vi "SetROI.vi"(8 "error in (no error)":errorcluster, 10 "fullWidth?":bool, 11 "Config In":T1 {"Hardware Configuration"."Lasers Configuration"."SettingValues"."785 Power" format="%.1f"; "Hardware Configuration"."Lasers Configuration"."SettingValues"."647 Power" format="%.1f"; "Hardware Configuration"."Lasers Configuration"."SettingValues"."561 Power" format="%.1f"}) -> (0 "error out":errorcluster, 3 "Config Out":T1 {"Hardware Configuration"."Lasers Configuration"."SettingValues"."785 Power" format="%.1f"; "Hardware Configuration"."Lasers Configuration"."SettingValues"."647 Power" format="%.1f"; "Hardware Configuration"."Lasers Configuration"."SettingValues"."561 Power" format="%.1f"})   [LabVIEW 2020]
uses:
  Settings/System Running Settings.ctl
  Support/Hardware Configuration.ctl
  Support/Camera Configuration.ctl
  controls/ROI.ctl
  D:/Daguan/Development/RM21-MMicrosopeSource/HardwareAdapter/Camera/Dependencies/PVCamNET.dll
  Dependencies/PVCamNET.dll
  <vilib>/vision/Image Controls.llb/IMAQ Image.ctl
  D:/Daguan/Development/RM21-MMicrosopeSource/HardwareAdapter/Lasers/Dependencies/Oxxius_Boxx.dll
  Lasers/Dependencies/Oxxius_Boxx.dll
  Logging/Logging Configuration.ctl
  controls/DeviceStatusCtl.ctl
  controls/CallBack Refs.ctl
  Logging/Logging.lvlib
  Settings/Settings.lvlib
panel:
  in  "Full CCD Height":u16
  in  "Full CCD Width":u16
  in  "Height":u16
  in  "Y":u16
  in  "Width":u16
  in  "X":u16
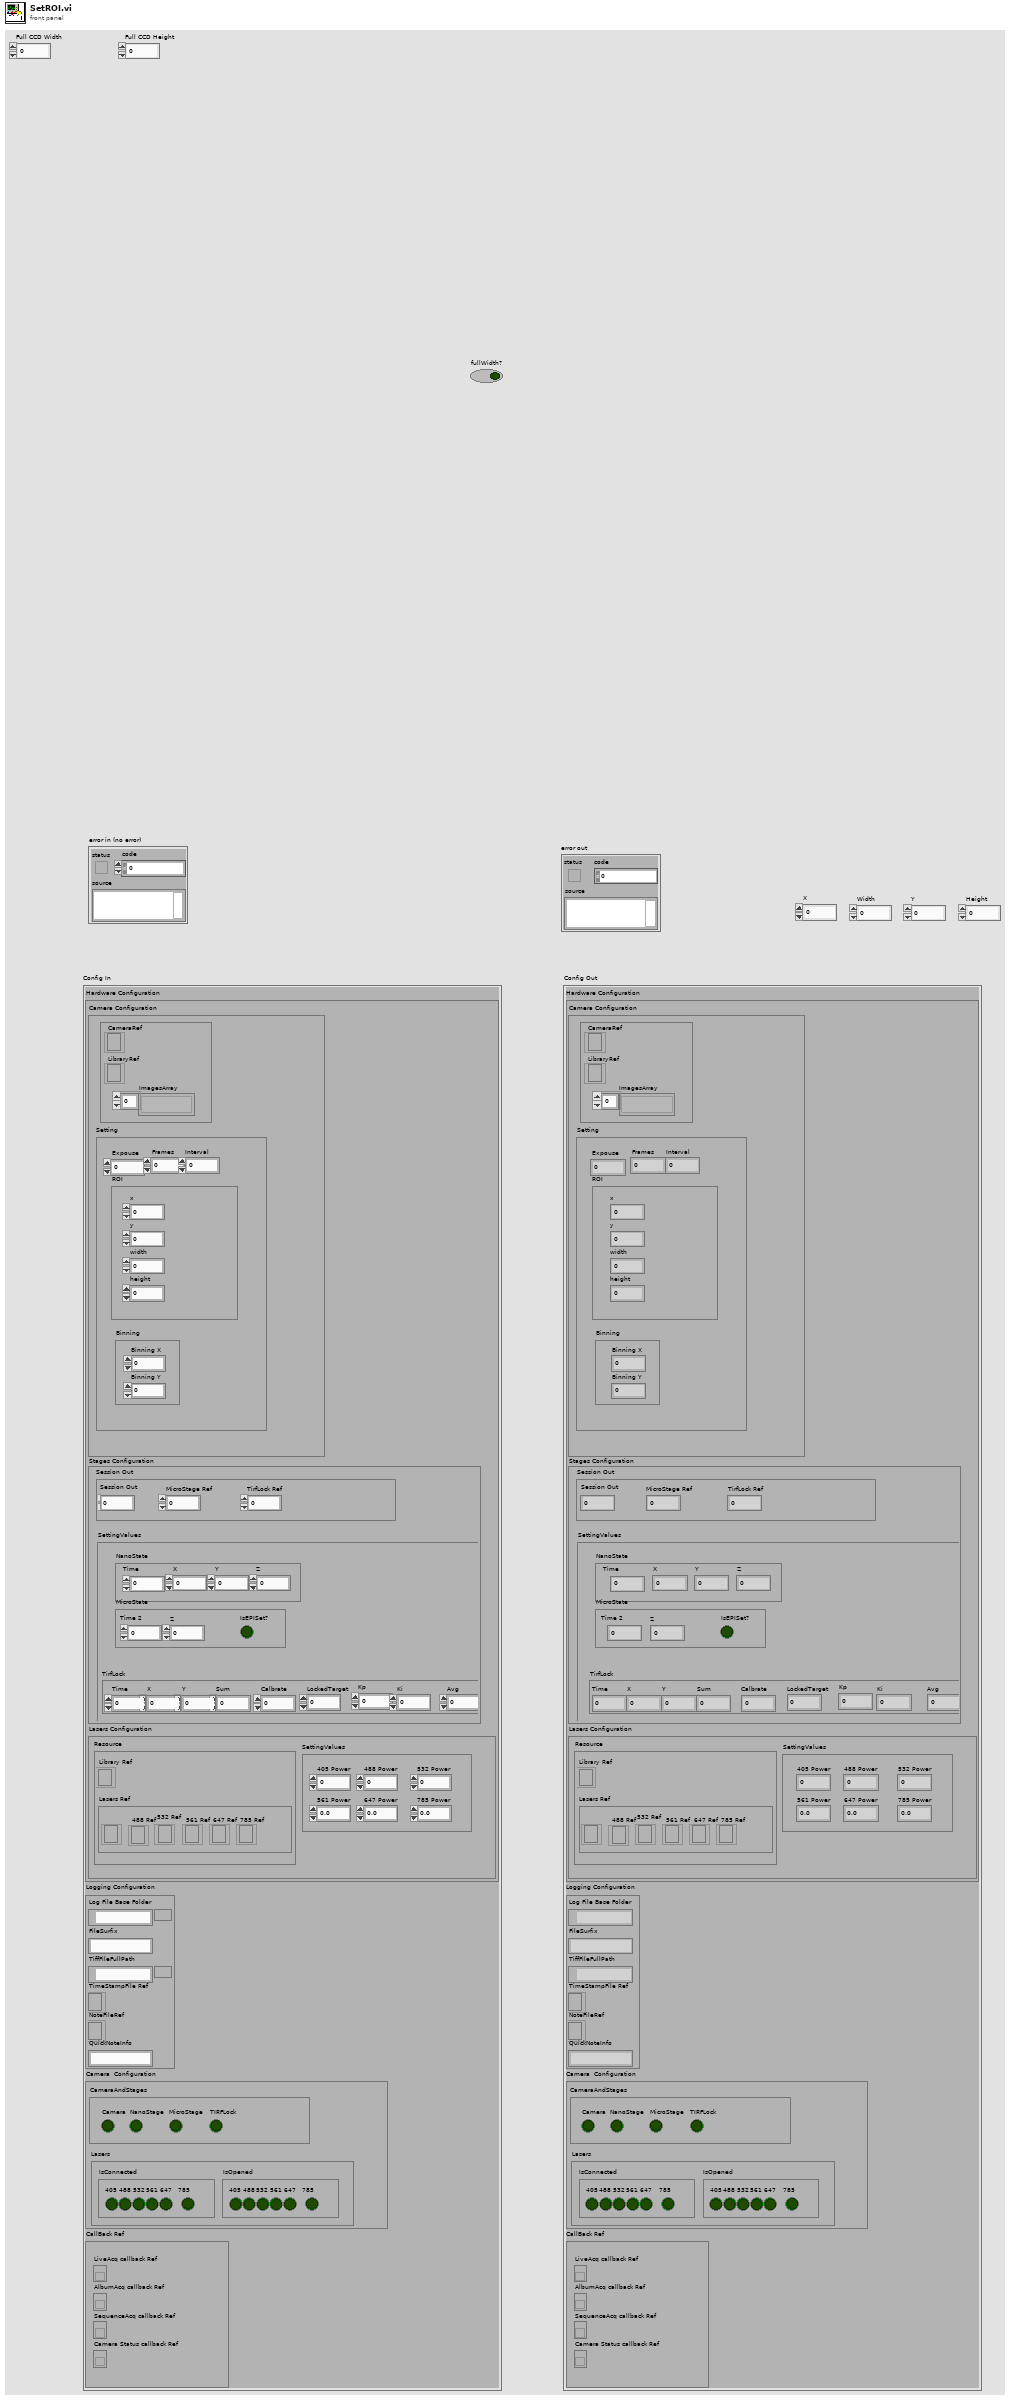
[diagram p1: front panel]
types:
  T1 = typedef "Settings.lvlib/System Running Settings.ctl" = cluster{"Hardware Configuration":T2, "Logging Configuration":T6, "HardWare Status":cluster{"CameraAndStages":T7, "Lasers":cluster{"IsConnected":cluster{"405":bool, "488":bool, "532":bool, "561":bool, "647":bool, "785":bool}, "IsOpened":cluster{"405":bool, "488":bool, "532":bool, "561":bool, "647":bool, "785":bool}}}, "CallBack Ref":T8}
  T2 = typedef "Hardware Configuration.ctl" = cluster{"Camera Configuration":T3, "Stages Configuration":cluster{"Resource":cluster{"NanoStage Ref":i32, "MicroStage Ref":i32, "TirfLock Ref":i32}, "SettingValues":cluster{"NanoState":cluster{"Time":dbl, "X":dbl, "Y":dbl, "Z":dbl}, "MicroState":cluster{"Time 2":dbl, "Z":dbl, "IsEPISet?":bool}, "TirfLock":cluster{"Time":dbl, "X":dbl, "Y":dbl, "Sum":dbl, "Calbrate":dbl, "LockedTarget":dbl, "Kp":dbl, "Ki":dbl, "Avg":dbl}}}, "Lasers Configuration":cluster{"SettingValues":cluster{"405 Power":sgl, "488 Power":sgl, "532 Power":sgl, "561 Power":sgl, "647 Power":sgl, "785 Power":sgl}, "Resource":cluster{"Library Ref":refnum<k24>, "Lasers Ref":cluster{"405 Ref":refnum<k24>, "488 Ref":refnum<k24>, "532 Ref":refnum<k24>, "561 Ref":refnum<k24>, "647 Ref":refnum<k24>, "785 Ref":refnum<k24>}}}}
  T3 = typedef "Camera Configuration.ctl" = cluster{"Setting":cluster{"Expouse":dbl, "Frames":dbl, "Interval":dbl, "ROI":T4, "Binning":cluster{"Binning X":dbl, "Binning Y":dbl}}, "Resource":cluster{"CameraRef":refnum<k24>, "LibraryRef":refnum<k24>, "ImagesArray":T5[]}}
  T4 = typedef "ROI.ctl" = cluster{"x":dbl, "y":dbl, "width":dbl, "height":dbl}
  T5 = typedef "IMAQ Image.ctl" = refnum<image>
  T6 = typedef "Logging.lvlib/Logging Configuration.ctl" = cluster{"Log File Base Folder":path, "FileSurfix":string, "TiffFileFullPath":path, "TimeStampFile Ref":refnum<file>, "NoteFileRef":refnum<file>, "QuickNoteInfo":string}
  T7 = typedef "DeviceStatusCtl.ctl" = cluster{"Camera":bool, "NanoStage":bool, "MicroStage":bool, "TIRFLock":bool}
  T8 = typedef "CallBack Refs.ctl" = cluster{"LiveAcq callback Ref":refnum<k27>, "AlbumAcq callback Ref":refnum<k27>, "SequenceAcq callback Ref":refnum<k27>, "Camera Status callback Ref":refnum<k27>}
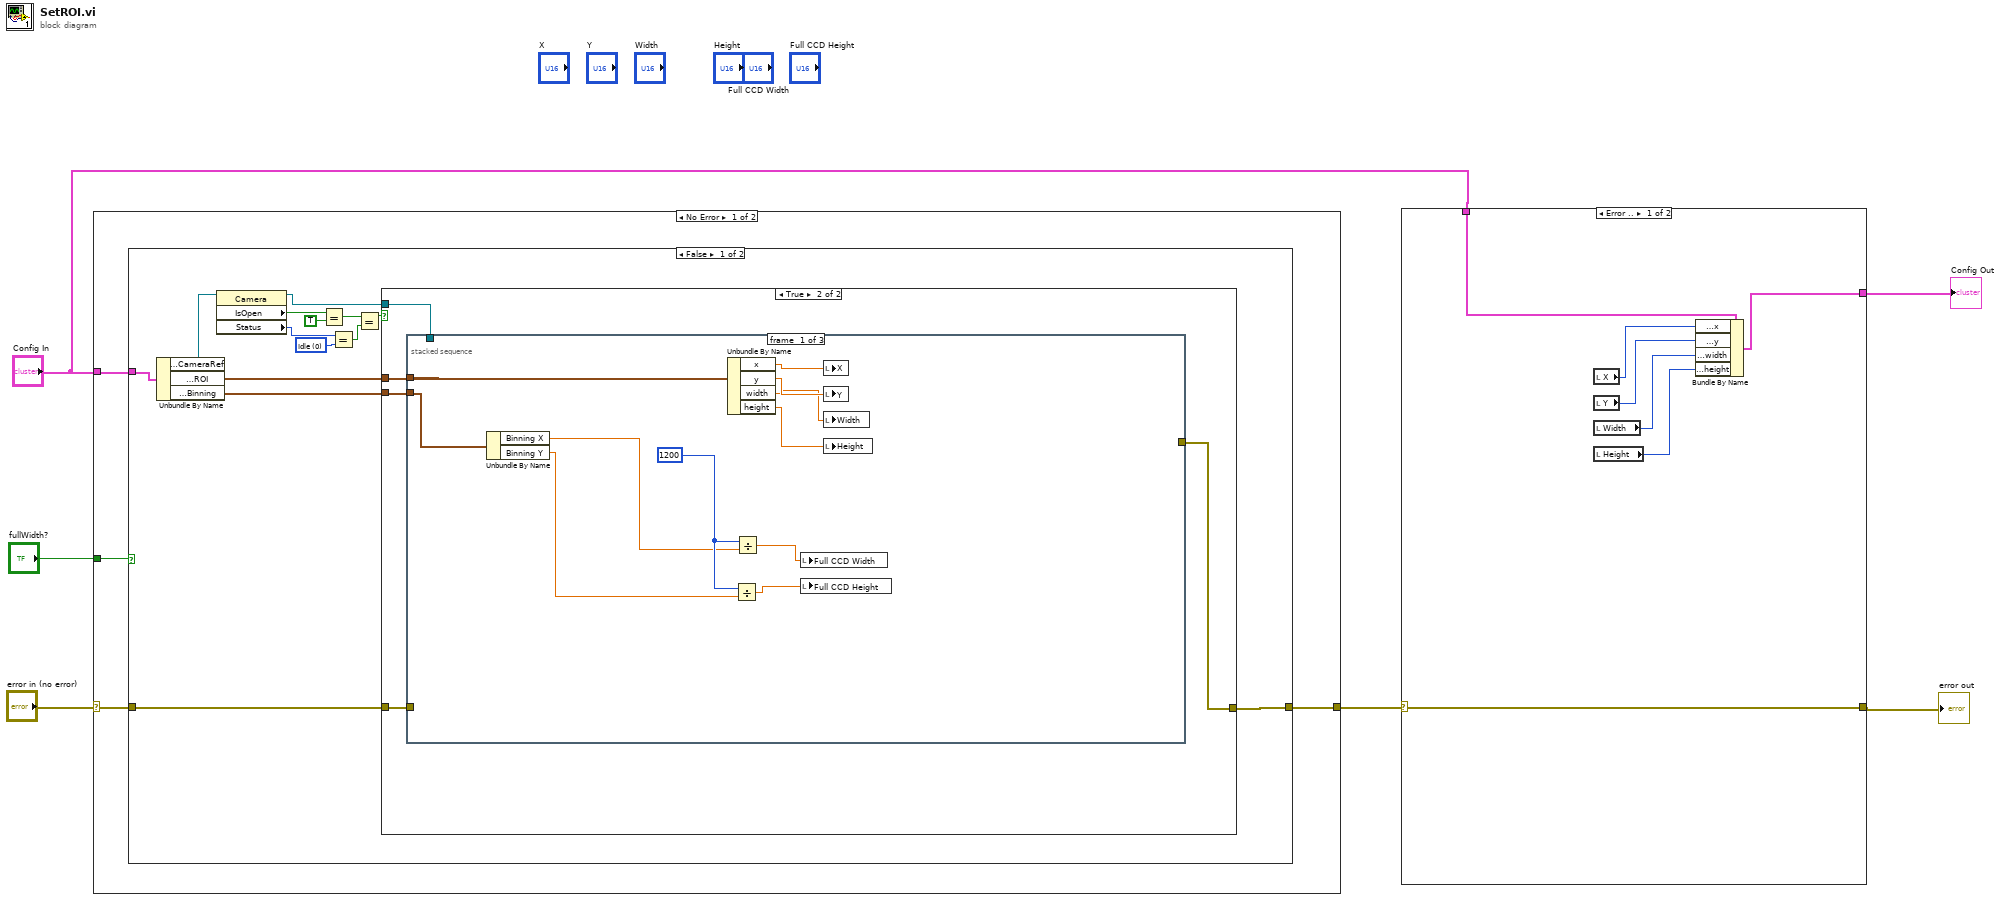
[diagram p0: block diagram]
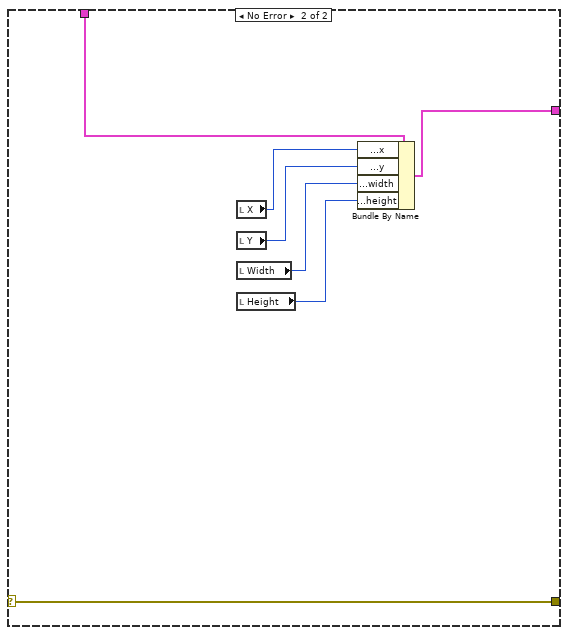
[diagram p2: hidden frame]
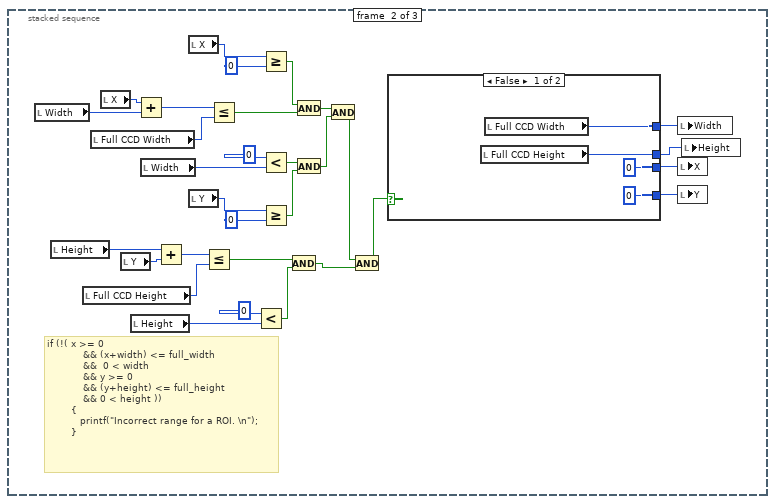
[diagram p4: hidden frame]
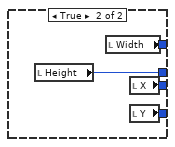
[diagram p5: hidden frame]
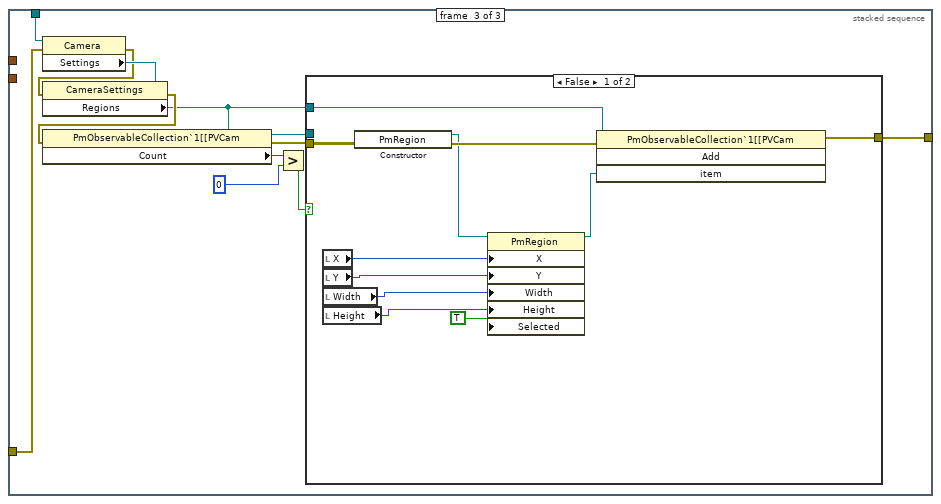
[diagram p6: hidden frame]
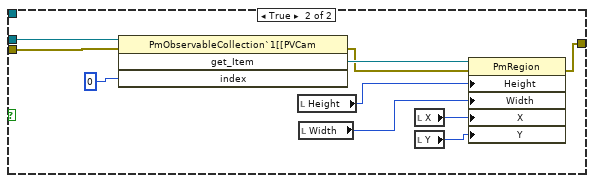
[diagram p7: hidden frame]
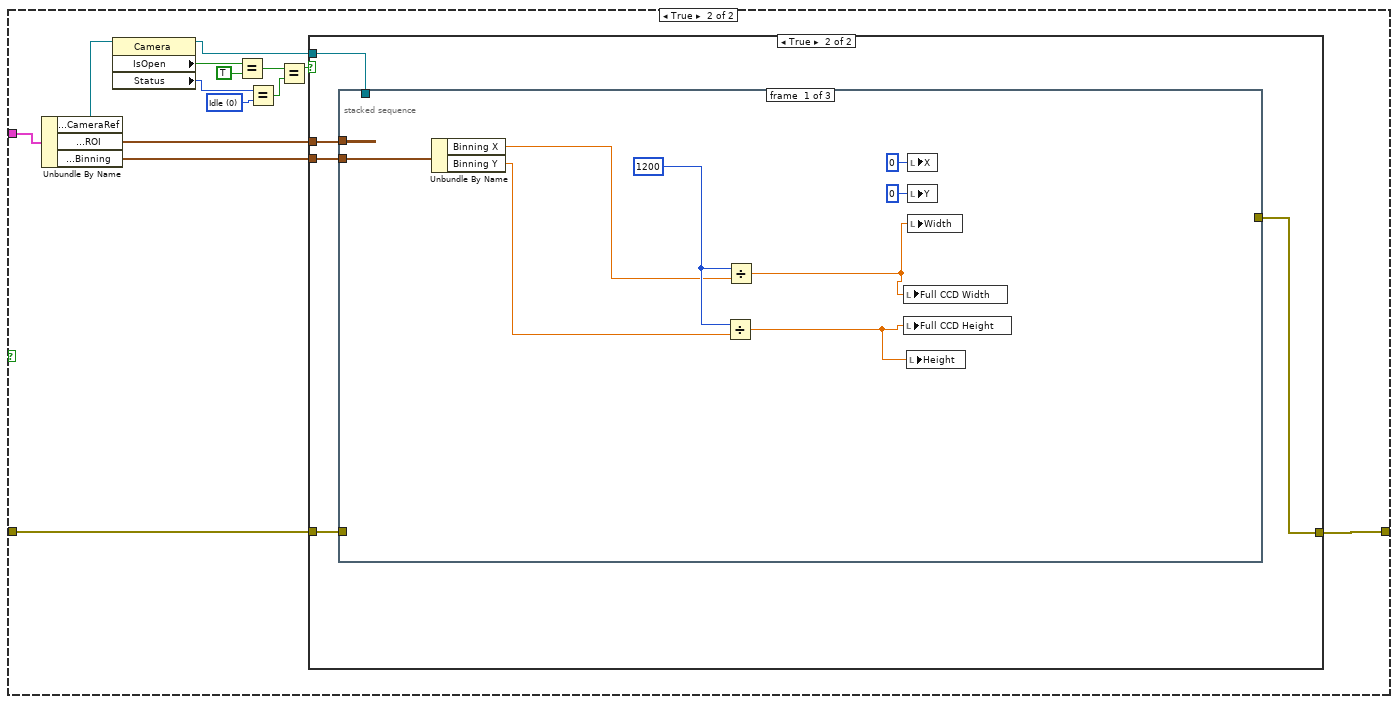
[diagram p8: hidden frame]
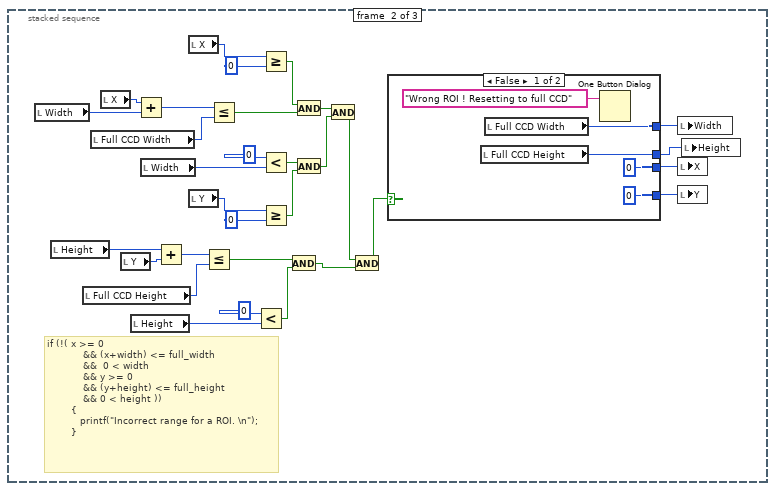
[diagram p10: hidden frame]
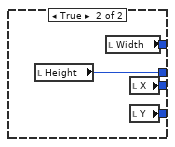
[diagram p11: hidden frame]
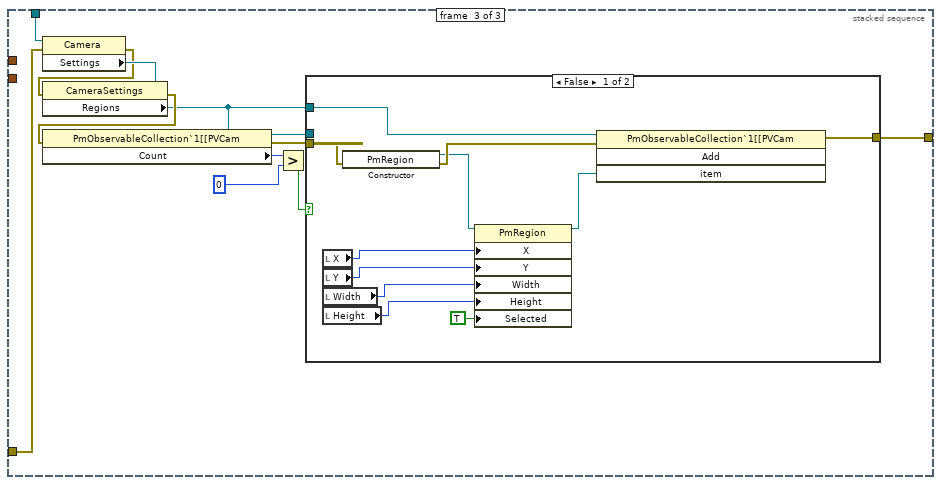
[diagram p12: hidden frame]
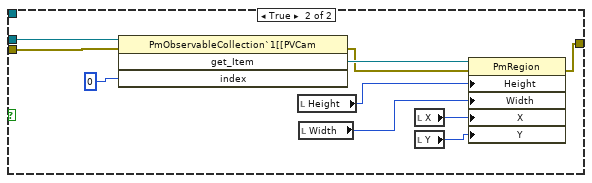
[diagram p13: hidden frame]
diagram:
  n1 = case shown="No Error" "error in (no error)" {
    selector: "error in (no error)" -> [w8 w215]
    tunnel: "fullWidth?" -> [w10 _]
    tunnel: "Config In" -> [w9 _]
    tunnel: [w7 w215] -> w4
    frame No Error {
      n2 = case shown="False" w10 {
        tunnel: w9 -> [w16 w119]
        tunnel: w8 -> [w14 w117]
        tunnel: [w13 w116] -> w7
        frame False {
          w23 = 0 items=["Idle", "Capturing"] ("Status")
          n3 = Unbundle By Name(w16) -> ("Hardware Configuration.Camera Configuration.Resource.CameraRef"=w12:refnum<k24>, "Hardware Configuration.Camera Configuration.Setting.ROI"=w15:T4, "Hardware Configuration.Camera Configuration.Setting.Binning"=w11:cluster{"Binning X":dbl, "Binning Y":dbl})
          n4 = property class="Camera"(reference=w12) -> (reference out=w17:refnum<k24>, "IsOpen"=w22:bool, "Status"=w24:i32)  [unwired: 1 in, 1 out]
          n5 = Equal?(x=w22, y=TRUE) -> (x = y?=w20:bool)
          n6 = Equal?(x=w24, y=w23) -> (x = y?=w19:bool)
          n7 = Equal?(x=w20, y=w19) -> (x = y?=w18:bool)
          n8 = case shown="True" w18 {
            tunnel: w17 -> [_ w30]
            tunnel: w15 -> [_ w29]
            tunnel: w14 -> [w25 w28]
            tunnel: [w25 w27] -> w13
            tunnel: w11 -> [_ w26]
            frame False {
            }
            frame True {
              n9 = stacked-sequence {
                tunnel: w29 -> [w41 _ _]
                tunnel: w30 -> [_ _ w92]
                tunnel: w28 -> [_ _ w86]
                tunnel: [_ _ w82] -> w27
                tunnel: w26 -> [w36 _ _]
                frame #0 {
                  w35 = u16 1200 ("Full CCD Width")
                  n10 = Unbundle By Name(w36) -> ("Binning X"=w34:dbl, "Binning Y"=w33:dbl)
                  n11 = Unbundle By Name(w41) -> ("x"=w40:dbl, "y"=w39:dbl, "width"=w38:dbl, "height"=w37:dbl)
                  n12 = Divide(x=w35, y=w33) -> (x/y=w31:dbl)
                  n13 = Divide(x=w35, y=w34) -> (x/y=w32:dbl)
                  n14 = local write "Full CCD Width"(w32) -> ()
                  n15 = local write "Full CCD Height"(w31) -> ()
                  n16 = local write "X"(w40) -> ()
                  n17 = local write "Y"(w39) -> ()
                  n18 = local write "Width"(w38) -> ()
                  n19 = local write "Height"(w37) -> ()
                }
                frame #1 {
                  # "if (!( x >= 0\n            && (x+width) <= full_width\n            &&  0 < width \n            && y >= 0\n            && (y+height) <= full_height\n            && 0 < height ))\n        {\n           printf(\"Incorrect range for a ROI. \\n\");\n        }"
                  n20 = local read "Width"() -> (w57:u16)
                  n21 = local read "Height"() -> (w55:u16)
                  n22 = local read "Full CCD Height"() -> (w51:u16)
                  n23 = local read "Full CCD Width"() -> (w53:u16)
                  n24 = local read "X"() -> (w58:u16)
                  n25 = local read "Y"() -> (w54:u16)
                  n26 = local read "Height"() -> (w46:u16)
                  n27 = Add(x=w58, y=w57) -> (x+y=w52:u16)
                  n28 = local read "Width"() -> (w49:u16)
                  n29 = Add(x=w55, y=w54) -> (x+y=w50:u16)
                  n30 = local read "X"() -> (w59:u16)
                  n31 = local read "Y"() -> (w56:u16)
                  n32 = Less Or Equal?(x=w50, y=w51) -> (x <= y?=w66:bool)
                  n33 = Less Or Equal?(x=w52, y=w53) -> (x <= y?=w69:bool)
                  n34 = Less?(x=u16 0 ("y"), y=w46) -> (x < y?=w65:bool)
                  n35 = Greater Or Equal?(x=w59, y=u16 0) -> (x >= y?=w70:bool)
                  n36 = Less?(x=u16 0 ("y"), y=w49) -> (x < y?=w68:bool)
                  n37 = Greater Or Equal?(x=w56, y=u16 0) -> (x >= y?=w67:bool)
                  n38 = And(x=w66, y=w65) -> (x .and. y?=w61:bool)
                  n39 = And(x=w70, y=w69) -> (x .and. y?=w64:bool)
                  n40 = And(x=w68, y=w67) -> (x .and. y?=w63:bool)
                  n41 = And(x=w64, y=w63) -> (x .and. y?=w62:bool)
                  n42 = And(x=w62, y=w61) -> (x .and. y?=w60:bool)
                  n43 = case shown="False" w60 {
                    tunnel: [w73 w80] -> w45
                    tunnel: [u16 0 ("X") w79] -> w42
                    tunnel: [u16 0 ("Y") w78] -> w43
                    tunnel: [w74 w77] -> w44
                    frame False {
                      n44 = local read "Full CCD Height"() -> (w74:u16)
                      n45 = local read "Full CCD Width"() -> (w73:u16)
                    }
                    frame True {
                      n46 = local read "Height"() -> (w77:u16)
                      n47 = local read "Width"() -> (w80:u16)
                      n48 = local read "X"() -> (w79:u16)
                      n49 = local read "Y"() -> (w78:u16)
                    }
                  }
                  n50 = local write "Width"(w45) -> ()
                  n51 = local write "X"(w42) -> ()
                  n52 = local write "Y"(w43) -> ()
                  n53 = local write "Height"(w44) -> ()
                }
                frame #2 {
                  n54 = property class="Camera"(reference=w92, error in=w86) -> (error out=w85:errorcluster, "Settings"=w91:refnum<k24>)  [unwired: 1 out]
                  n55 = property class="CameraSettings"(reference=w91, error in=w85) -> (error out=w84:errorcluster, "Regions"=w81:refnum<k24>)  [unwired: 1 out]
                  n56 = property class="PmObservableCollection`1[[PVCam"(reference=w81, error in=w84) -> (reference out=w87:refnum<k24>, error out=w83:errorcluster, "Count"=w90:i32)
                  n57 = Greater?(x=w90, y=0) -> (0:w88:bool)
                  n58 = case shown="False" w88 {
                    tunnel: w87 -> [_ w111]
                    tunnel: w83 -> [w95 w106]
                    tunnel: [w103 w104] -> w82
                    tunnel: w81 -> [w96 _]
                    frame False {
                      n59 = local read "X"() -> (w101:u16)
                      n60 = local read "Y"() -> (w100:u16)
                      n61 = local read "Width"() -> (w99:u16)
                      n62 = local read "Height"() -> (w98:u16)
                      n63 = constructor class="PmRegion"(error in=w95) -> (reference out=w93:refnum<k24>, error out=w94:errorcluster)  [unwired: 2 in, 1 out]
                      n64 = property class="PmRegion"(reference=w93, "X"=w101, "Y"=w100, "Width"=w99, "Height"=w98, "Selected"=TRUE) -> (reference out=w102:refnum<k24>)  [unwired: 1 in, 1 out]
                      n65 = invoke class="PmObservableCollection`1[[PVCam" method="Add"(reference=w96, error in=w94, "item"=w102) -> (error out=w103:errorcluster)  [unwired: 1 in, 3 out]
                    }
                    frame True {
                      n66 = invoke class="PmObservableCollection`1[[PVCam" method="get_Item"(reference=w111, error in=w106, "index"=0) -> (error out=w105:errorcluster, "get_Item"=w113:refnum<k24>)  [unwired: 1 in, 2 out]
                      n67 = local read "Height"() -> (w110:u16)
                      n68 = local read "Width"() -> (w109:u16)
                      n69 = local read "X"() -> (w108:u16)
                      n70 = local read "Y"() -> (w107:u16)
                      n71 = property class="PmRegion"(reference=w113, error in=w105, "Height"=w110, "Width"=w109, "X"=w108, "Y"=w107) -> (error out=w104:errorcluster)  [unwired: 1 out]
                    }
                  }
                }
              }
            }
          }
        }
        frame True {
          w126 = 0 items=["Idle", "Capturing"] ("Status")
          n72 = Unbundle By Name(w119) -> ("Hardware Configuration.Camera Configuration.Resource.CameraRef"=w115:refnum<k24>, "Hardware Configuration.Camera Configuration.Setting.ROI"=w118:T4, "Hardware Configuration.Camera Configuration.Setting.Binning"=w114:cluster{"Binning X":dbl, "Binning Y":dbl})
          n73 = property class="Camera"(reference=w115) -> (reference out=w120:refnum<k24>, "IsOpen"=w125:bool, "Status"=w127:i32)  [unwired: 1 in, 1 out]
          n74 = Equal?(x=w125, y=TRUE) -> (x = y?=w123:bool)
          n75 = Equal?(x=w127, y=w126) -> (x = y?=w122:bool)
          n76 = Equal?(x=w123, y=w122) -> (x = y?=w121:bool)
          n77 = case shown="True" w121 {
            tunnel: w120 -> [_ w133]
            tunnel: w118 -> [_ w132]
            tunnel: w117 -> [w128 w131]
            tunnel: [w128 w130] -> w116
            tunnel: w114 -> [_ w129]
            frame False {
            }
            frame True {
              n78 = stacked-sequence {
                tunnel: w132 -> [_ _ _]
                tunnel: w133 -> [_ _ w193]
                tunnel: w131 -> [_ _ w187]
                tunnel: [_ _ w183] -> w130
                tunnel: w129 -> [w136 _ _]
                frame #0 {
                  w139 = u16 1200 ("Full CCD Width")
                  n79 = Unbundle By Name(w136) -> ("Binning X"=w138:dbl, "Binning Y"=w137:dbl)
                  n80 = Divide(x=w139, y=w137) -> (x/y=w134:dbl)
                  n81 = Divide(x=w139, y=w138) -> (x/y=w135:dbl)
                  n82 = local write "Full CCD Width"(w135) -> ()
                  n83 = local write "Full CCD Height"(w134) -> ()
                  n84 = local write "Height"(w134) -> ()
                  n85 = local write "X"(u16 0 ("X")) -> ()
                  n86 = local write "Y"(u16 0 ("Y")) -> ()
                  n87 = local write "Width"(w135) -> ()
                }
                frame #1 {
                  # "if (!( x >= 0\n            && (x+width) <= full_width\n            &&  0 < width \n            && y >= 0\n            && (y+height) <= full_height\n            && 0 < height ))\n        {\n           printf(\"Incorrect range for a ROI. \\n\");\n        }"
                  n88 = local read "Width"() -> (w157:u16)
                  n89 = local read "Height"() -> (w155:u16)
                  n90 = local read "Full CCD Height"() -> (w151:u16)
                  n91 = local read "Full CCD Width"() -> (w153:u16)
                  n92 = local read "X"() -> (w158:u16)
                  n93 = local read "Y"() -> (w154:u16)
                  n94 = local read "Height"() -> (w146:u16)
                  n95 = Add(x=w158, y=w157) -> (x+y=w152:u16)
                  n96 = local read "Width"() -> (w149:u16)
                  n97 = Add(x=w155, y=w154) -> (x+y=w150:u16)
                  n98 = local read "X"() -> (w159:u16)
                  n99 = local read "Y"() -> (w156:u16)
                  n100 = Less Or Equal?(x=w150, y=w151) -> (x <= y?=w166:bool)
                  n101 = Less Or Equal?(x=w152, y=w153) -> (x <= y?=w169:bool)
                  n102 = Less?(x=u16 0 ("y"), y=w146) -> (x < y?=w165:bool)
                  n103 = Greater Or Equal?(x=w159, y=u16 0) -> (x >= y?=w170:bool)
                  n104 = Less?(x=u16 0 ("y"), y=w149) -> (x < y?=w168:bool)
                  n105 = Greater Or Equal?(x=w156, y=u16 0) -> (x >= y?=w167:bool)
                  n106 = And(x=w166, y=w165) -> (x .and. y?=w161:bool)
                  n107 = And(x=w170, y=w169) -> (x .and. y?=w164:bool)
                  n108 = And(x=w168, y=w167) -> (x .and. y?=w163:bool)
                  n109 = And(x=w164, y=w163) -> (x .and. y?=w162:bool)
                  n110 = And(x=w162, y=w161) -> (x .and. y?=w160:bool)
                  n111 = case shown="False" w160 {
                    tunnel: [w174 w181] -> w145
                    tunnel: [u16 0 ("X") w180] -> w142
                    tunnel: [u16 0 ("Y") w179] -> w143
                    tunnel: [w175 w178] -> w144
                    frame False {
                      n112 = local read "Full CCD Height"() -> (w175:u16)
                      n113 = local read "Full CCD Width"() -> (w174:u16)
                      n114 = One Button Dialog(message="Wrong ROI ! Resetting to full CCD") -> ()  [unwired: 1 in, 1 out]
                    }
                    frame True {
                      n115 = local read "Height"() -> (w178:u16)
                      n116 = local read "Width"() -> (w181:u16)
                      n117 = local read "X"() -> (w180:u16)
                      n118 = local read "Y"() -> (w179:u16)
                    }
                  }
                  n119 = local write "Width"(w145) -> ()
                  n120 = local write "X"(w142) -> ()
                  n121 = local write "Y"(w143) -> ()
                  n122 = local write "Height"(w144) -> ()
                }
                frame #2 {
                  n123 = property class="Camera"(reference=w193, error in=w187) -> (error out=w186:errorcluster, "Settings"=w192:refnum<k24>)  [unwired: 1 out]
                  n124 = property class="CameraSettings"(reference=w192, error in=w186) -> (error out=w185:errorcluster, "Regions"=w182:refnum<k24>)  [unwired: 1 out]
                  n125 = property class="PmObservableCollection`1[[PVCam"(reference=w182, error in=w185) -> (reference out=w188:refnum<k24>, error out=w184:errorcluster, "Count"=w191:i32)
                  n126 = Greater?(x=w191, y=0) -> (0:w189:bool)
                  n127 = case shown="False" w189 {
                    tunnel: w188 -> [_ w212]
                    tunnel: w184 -> [w196 w207]
                    tunnel: [w203 w205] -> w183
                    tunnel: w182 -> [w204 _]
                    frame False {
                      n128 = local read "X"() -> (w201:u16)
                      n129 = local read "Y"() -> (w200:u16)
                      n130 = local read "Width"() -> (w199:u16)
                      n131 = local read "Height"() -> (w198:u16)
                      n132 = constructor class="PmRegion"(error in=w196) -> (reference out=w194:refnum<k24>, error out=w195:errorcluster)  [unwired: 2 in, 1 out]
                      n133 = property class="PmRegion"(reference=w194, "X"=w201, "Y"=w200, "Width"=w199, "Height"=w198, "Selected"=TRUE) -> (reference out=w202:refnum<k24>)  [unwired: 1 in, 1 out]
                      n134 = invoke class="PmObservableCollection`1[[PVCam" method="Add"(reference=w204, error in=w195, "item"=w202) -> (error out=w203:errorcluster)  [unwired: 1 in, 3 out]
                    }
                    frame True {
                      n135 = invoke class="PmObservableCollection`1[[PVCam" method="get_Item"(reference=w212, error in=w207, "index"=0) -> (error out=w206:errorcluster, "get_Item"=w214:refnum<k24>)  [unwired: 1 in, 2 out]
                      n136 = local read "Height"() -> (w211:u16)
                      n137 = local read "Width"() -> (w210:u16)
                      n138 = local read "X"() -> (w209:u16)
                      n139 = local read "Y"() -> (w208:u16)
                      n140 = property class="PmRegion"(reference=w214, error in=w206, "Height"=w211, "Width"=w210, "X"=w209, "Y"=w208) -> (error out=w205:errorcluster)  [unwired: 1 out]
                    }
                  }
                }
              }
            }
          }
        }
      }
    }
    frame Error {
    }
  }
  n141 = case shown="Error .." w4 {
    selector: w4 -> [w222 w229]
    tunnel: [w222 w229] -> w3
    tunnel: "Config In" -> [w221 w228]
    tunnel: [w216 w223] -> w1
    frame Error {
      n142 = local read "X"() -> (w220:u16)
      n143 = local read "Y"() -> (w219:u16)
      n144 = local read "Width"() -> (w218:u16)
      n145 = local read "Height"() -> (w217:u16)
      n146 = Bundle By Name(cluster=w221, "Hardware Configuration.Camera Configuration.Setting.ROI.x"=w220, "Hardware Configuration.Camera Configuration.Setting.ROI.y"=w219, "Hardware Configuration.Camera Configuration.Setting.ROI.width"=w218, "Hardware Configuration.Camera Configuration.Setting.ROI.height"=w217) -> (w216:T1)
    }
    frame No Error {
      n147 = local read "X"() -> (w227:u16)
      n148 = local read "Y"() -> (w226:u16)
      n149 = local read "Width"() -> (w225:u16)
      n150 = local read "Height"() -> (w224:u16)
      n151 = Bundle By Name(cluster=w228, "Hardware Configuration.Camera Configuration.Setting.ROI.x"=w227, "Hardware Configuration.Camera Configuration.Setting.ROI.y"=w226, "Hardware Configuration.Camera Configuration.Setting.ROI.width"=w225, "Hardware Configuration.Camera Configuration.Setting.ROI.height"=w224) -> (w223:T1)
    }
  }
  "error out" <- w3
  "Config Out" <- w1
